vi "Configure VIs for Execution.vi"   [LabVIEW 2017]
types:
  T1 = cluster{"Status Message":refnum<data-value>, "Progress":refnum<data-value>, "Stop":refnum<data-value>}
  T2 = enum16{"Share clones between instances", "Preallocate clone for each instance"}
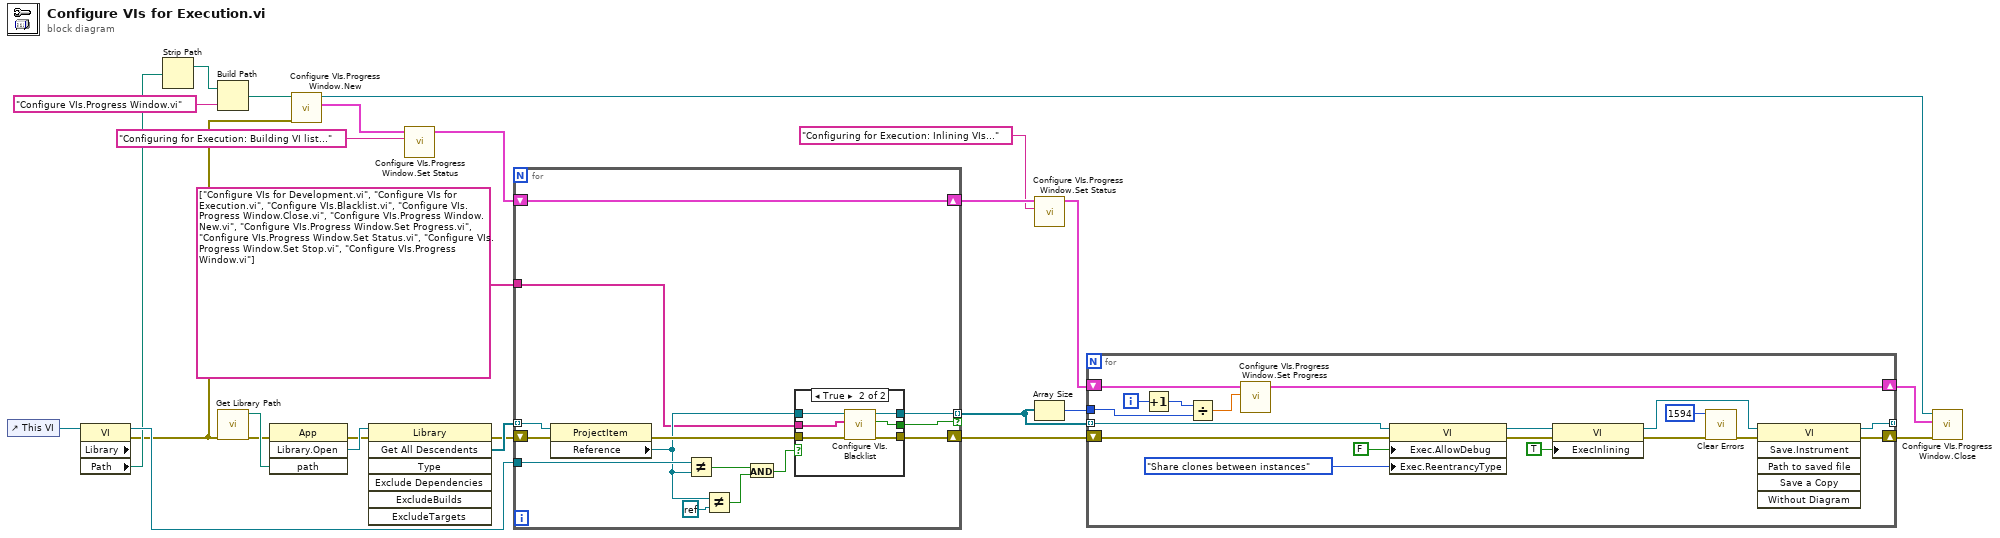
[diagram p0: block diagram]
diagram:
  n1 = control-ref of="This VI"() -> (w26:refnum<vi>)
  n2 = property class="VI" props=["Library", "Path"](reference=w26) -> (reference out=w25:refnum<vi>, error out=w7:errorcluster, "Path"=w8:path)  [unwired: 1 in, 1 out]
  n3 = Strip Path(path=w8) -> (stripped path=w23:path)  [unwired: 1 out]
  n4 = Build Path(base path=w23, name or relative path="Configure VIs.Progress Window.vi") -> (appended path=w22:path)
  n5 = call "Get Library Path.vi"("error in (no error)"=w7) -> ("error out"=w3:errorcluster, "Path"=w6:path)  [unwired: 9 in]
  n6 = invoke class="App" method="Library.Open"(error in=w3, "path"=w6) -> (error out=w2:errorcluster, "Open Library"=w5:refnum<vi>)  [unwired: 2 in, 2 out]
  n7 = call "Configure VIs.Progress Window.New.vi"("error in (no error)"=w7, "VI path"=w22) -> ("DVRs"=w17:T1, "VI refnum"=w10:refnum<vi>)  [unwired: 7 in, 1 out]
  n8 = invoke class="Library" method="Get All Descendents"(reference=w5, error in=w2) -> (error out=w1:errorcluster, "All Descendents"=w4:refnum<vi>[])  [unwired: 5 in, 5 out]
  n9 = call "Configure VIs.Progress Window.Set Status.vi"("Status Message"="Configuring for Execution: Building VI list..." ("data value"), "DVRs in"=w17) -> ("DVRs out"=w18:T1)  [unwired: 8 in, 1 out]
  n10 = for {
    tunnel: w4 -> [w40] mode=indexing
    tunnel: [w39] -> w20 mode=indexing if=w38
    tunnel: w25 -> [w36]
    shift-right: [w34] -> w24
    shift-left: w1 -> [w33]
    shift-right: [w28] -> w15
    shift-left: w18 -> [w28]
    tunnel: string[] ["Configure VIs for Development.vi", "Configure VIs for Execution.vi", "Configure VIs.Blacklist.vi", "Configure VIs.Progress Window.Close.vi", "Configure VIs.Progress Window.New.vi", "Configure VIs.Progress Window.Set Progress.vi", "Configure VIs.Progress Window.Set Status.vi", "Configure VIs.Progress Window.Set Stop.vi", "Configure VIs.Progress Window.vi"] ("Blacklist VIs") -> [w27]
    n11 = property class="ProjectItem"(reference=w40, error in=w33) -> (error out=w32:errorcluster, "Reference"=w29:refnum<vi>)  [unwired: 1 out]
    n12 = Not Equal?(x=w36, y=w29) -> (x != y?=w35:bool)
    n13 = Not Equal?(x=w29, y=refnum<k0> refnum) -> (x != y?=w31:bool)
    n14 = And(x=w35, y=w31) -> (x .and. y?=w30:bool)
    n15 = case shown="True" w30 {
      selector: w30 -> [w42 _]
      tunnel: [w43 w47] -> w39
      tunnel: [w42 w45] -> w38
      tunnel: w29 -> [w43 w49]
      tunnel: [w41 w46] -> w34
      tunnel: w32 -> [w41 w48]
      tunnel: w27 -> [_ w44]
      frame False {
      }
      frame True {
        n16 = call "Configure VIs.Blacklist.vi"("error in (no error)"=w48, "Blacklist VIs"=w44, "VI reference in"=w49) -> ("error out"=w46:errorcluster, "valid?"=w45:bool, "VI reference out"=w47:refnum<vi>)  [unwired: 6 in]
      }
    }
  }
  n17 = call "Configure VIs.Progress Window.Set Status.vi"("Status Message"="Configuring for Execution: Inlining VIs..." ("data value"), "DVRs in"=w15) -> ("DVRs out"=w14:T1)  [unwired: 8 in, 1 out]
  n18 = Array Size(array=w20) -> (size(s)=w19:i32)
  n19 = for {
    tunnel: w20 -> [w58] mode=indexing
    tunnel: [w64] -> _ mode=indexing
    shift-right: [w65] -> w11
    shift-left: w24 -> [w57]
    tunnel: w19 -> [w66]
    shift-right: [w61] -> w12
    shift-left: w14 -> [w63]
    i -> [w68]
    n20 = Increment(x=w68) -> (x+1=w67:i32)
    n21 = Divide(x=w67, y=w66) -> (x/y=w62:dbl)
    n22 = call "Configure VIs.Progress Window.Set Progress.vi"("Progress"=w62, "DVRs in"=w63) -> ("DVRs out"=w61:T1)  [unwired: 8 in, 1 out]
    n23 = property class="VI"(reference=w58, error in=w57, "Exec.AllowDebug"=FALSE ("Execution:Allow Debugging"), "Exec.ReentrancyType"=T2."Share clones between instances" ("Execution:Reentrancy Type")) -> (reference out=w52:refnum<vi>, error out=w53:errorcluster)
    n24 = property class="VI"(reference=w52, error in=w53, "ExecInlining"=TRUE ("Execution:Inline SubVI")) -> (reference out=w51:refnum<vi>, error out=w54:errorcluster)
    n25 = call <vilib>:"Clear Errors.vi"("error in (no error)"=w54, "specific error code to clear (0: all)"=1594) -> ("error out"=w50:errorcluster)  [unwired: 4 in, 1 out]
    n26 = invoke class="VI" method="Save.Instrument"(reference=w51, error in=w50) -> (reference out=w64:refnum<vi>, error out=w65:errorcluster)  [unwired: 4 in, 4 out]
  }
  n27 = call "Configure VIs.Progress Window.Close.vi"("error in (no error)"=w11, "DVRs in"=w12, "VI refnum"=w10) -> ()  [unwired: 8 in, 1 out]
